vi "DIGIT_5122_Run_And_Fetch.vi"(8 "error in (no error)":errorcluster, 11 "instrument handle":refnum<k15> caption="instrument handle in") -> (0 "error out":errorcluster, 1 "wfm info":T1(array[cluster]) {"reserved2" format="%.2f"; "reserved1" format="%.2f"; "offset" format="%^.3e"; "gain" format="%^.3e"; "xIncrement" format="%^.3e"; "relativeInitialX" format="%^.3e"; "absoluteInitialX" format="%^.3e"}, 2 "dataset":i16[][](array[numeric]), 3 "instrument handle out":refnum<k15>)   [LabVIEW 2024]
doc: "Monitors the status information indicating whether an acquisition is in progress, complete, or unknown.\nWhen the acquisition is completed, retrieves data from multiple channels and records.\nReturns a two-dimensional array of binary 16-bit waveforms."
uses:
  <instrlib>/niScope/Acquire/Fetch/niScope Multi Fetch Binary 16.vi
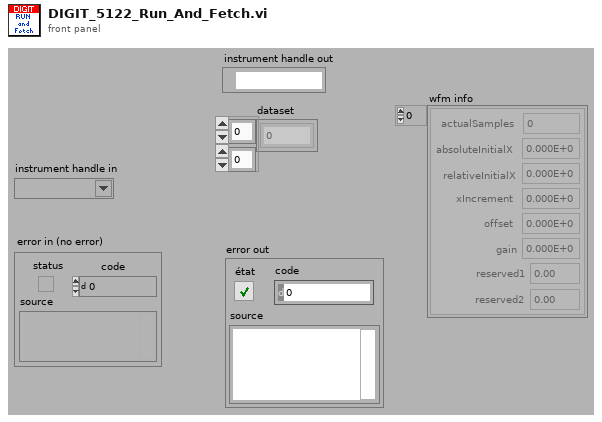
[diagram p1: front panel]
types:
  T1 = cluster{"actualSamples":i32, "absoluteInitialX":dbl, "relativeInitialX":dbl, "xIncrement":dbl, "offset":dbl, "gain":dbl, "reserved1":dbl, "reserved2":dbl}[]
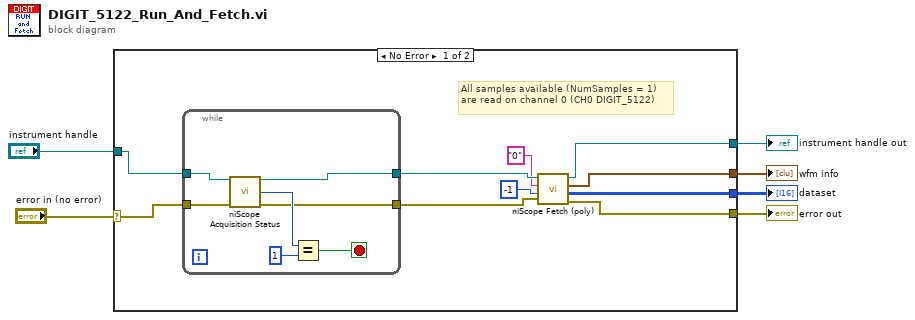
[diagram p0: block diagram]
diagram:
  n1 = case shown="No Error" "error in (no error)" {
    selector: "error in (no error)" -> [w13 w24]
    tunnel: "instrument handle" -> [w14 _]
    tunnel: [w12 _] -> w4
    tunnel: [w11 w24] -> w3
    tunnel: [w10 _] -> w2
    tunnel: [w7 _] -> w1
    frame No Error {
      # "All samples available (NumSamples = 1)\nare read on channel 0 (CH0 DIGIT_5122)"
      n2 = while {
        tunnel: w14 -> [w20]
        tunnel: [w21] -> w16
        tunnel: w13 -> [w19]
        tunnel: [w18] -> w15
        stop <- w17 stop-if-true
        n3 = call <instrlib>:"niScope Acquisition Status.vi"("instrument handle"=w20, "error in"=w19) -> ("instrument handle out"=w21:refnum<k15>, "acquisition status"=w23:i32, "error out"=w18:errorcluster)  [unwired: 11 in]
        n4 = Equal?(x=w23, y=1) -> (x = y?=w17:bool)
      }
      n5 = call-poly <instrlib>:"niScope Fetch (poly).vi"("error in"=w15, "numSamples"=-1, "channels"="0", "instrument handle"=w16) -> ("error out"=w11:errorcluster, "wfm"=w12:i16[][], "wfm info"=w7:T1, "instrument handle out"=w10:refnum<k15>)  [unwired: 4 in]
    }
    frame Error {
    }
  }
  "error out" <- w3
  "dataset" <- w4
  "instrument handle out" <- w2
  "wfm info" <- w1
